vi "5.vi"(2 "逆运动学输入":dbl[](array[numeric])=[0.2, 0.0, 0.3], 3 "123":dbl[](array[numeric]), 4 "机械臂末端姿态":dbl[][](array[numeric])) -> (0 "1235b":dbl[](array[numeric]), 1 "1235a":dbl[](array[numeric]))   [LabVIEW 2014]
uses:
  <vilib>/Utility/file.llb/Read From Spreadsheet File (DBL).vi
panel:
  out "t52":dbl
  out "t6":dbl
  out "t5":dbl
  out "t4":dbl
  out "angle33":dbl
  out "angle32":dbl
  out "angle52":dbl
  out "3角度输出":dbl[](array[numeric])
  out "角度/弧度":dbl
  out "弧度/角度":dbl
  out "az":dbl=1.0
  out "ay":dbl
  out "ax":dbl
  out "angle6":dbl
  out "angle5":dbl
  out "angle4":dbl
  out "angle3":dbl
  out "angle2":dbl
  out "angle1":dbl
  out "逆运动学输出":dbl[](array[numeric])=[0.0, 90.0, 0.0, 0.0, -90.0, -0.0] format="%#.3f"
  in  "机械臂臂长":dbl[](array[numeric])=[558.0, 764.0, 993.0, 420.0]
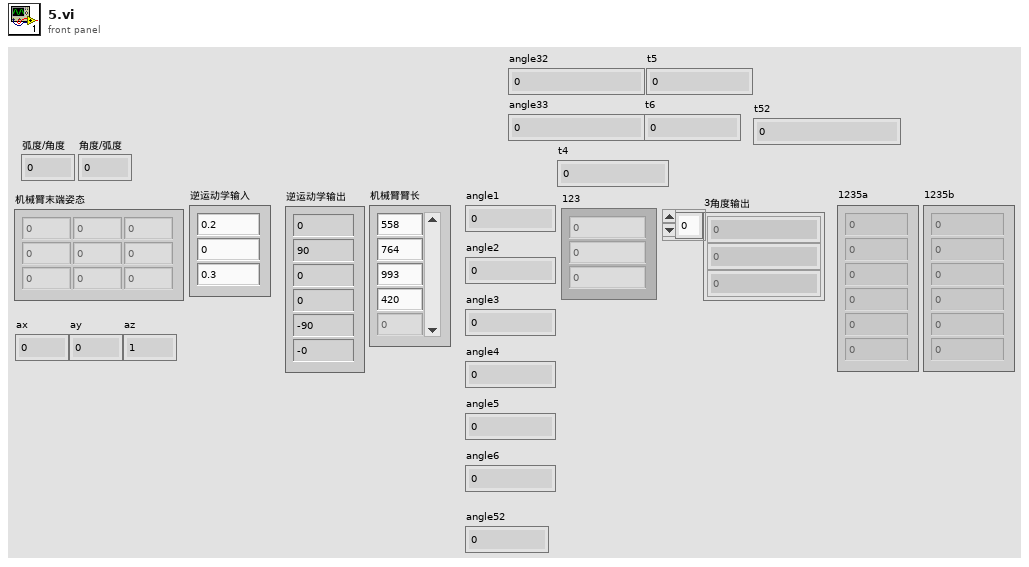
[diagram p1: front panel]
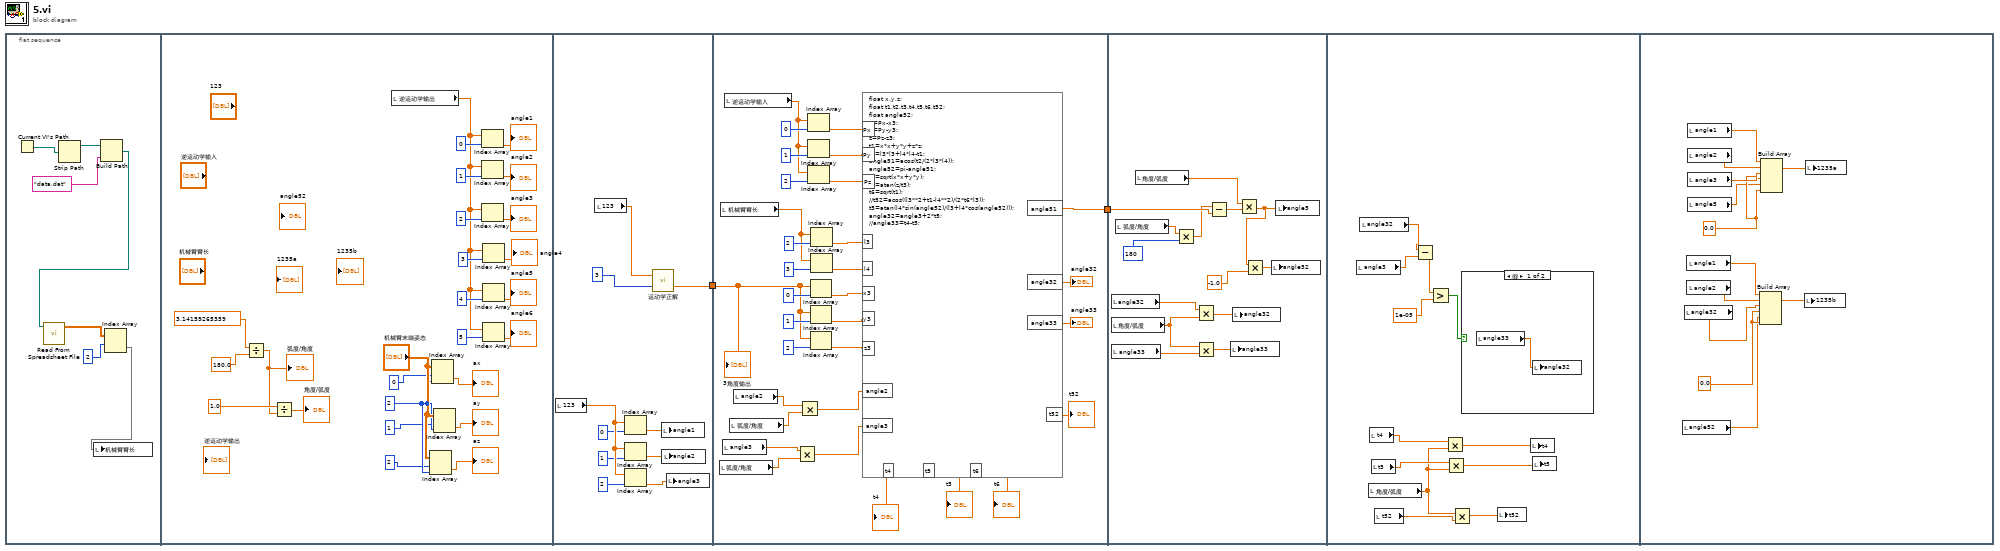
[diagram p0: block diagram]
diagram:
  n1 = flat-sequence {
    tunnel: [w44] -> w1
    tunnel: [w58] -> w2
    tunnel: w1 -> [w70]
    tunnel: w2 -> [w87]
    frame #0 {
      n2 = Current VI's Path() -> (path=w6:path)
      n3 = Strip Path(path=w6) -> (stripped path=w5:path)  [unwired: 1 out]
      n4 = Build Path(base path=w5, name or relative path="data.dat") -> (appended path=w3:path)
      n5 = call-poly <vilib>:"Read From Spreadsheet File.vi"("file path (dialog if empty)"=w3) -> ("all rows"=w9:dbl[][])  [unwired: 6 in, 4 out]
      n6 = Index Array(array=w9, index (row)=2) -> (element=w8:dbl[])  [unwired: 1 in]
      n7 = local write "机械臂臂长"(w8) -> ()
    }
    frame #1 {
      w19 = 2
      n8 = Divide(x=3.14159265359, y=180.0) -> (x/y=w11:dbl)
      "弧度/角度" <- w11
      n9 = Divide(x=1.0, y=w11) -> (x/y=→"角度/弧度":dbl)
      n10 = local read "逆运动学输出"() -> (w23:dbl[])
      n11 = Index Array(array="机械臂末端姿态", index (row)=2, index (col)=w19) -> (element=→"az":dbl)
      n12 = Index Array(array="机械臂末端姿态", index (row)=0, index (col)=w19) -> (element=→"ax":dbl)
      n13 = Index Array(array="机械臂末端姿态", index (row)=1, index (col)=w19) -> (element=→"ay":dbl)
      n14 = Index Array(array=w23, index=0) -> (element=→"angle1":dbl)
      n15 = Index Array(array=w23, index=1) -> (element=→"angle2":dbl)
      n16 = Index Array(array=w23, index=2) -> (element=→"angle3":dbl)
      n17 = Index Array(array=w23, index=3) -> (element=→"angle4":dbl)
      n18 = Index Array(array=w23, index=4) -> (element=→"angle5":dbl)
      n19 = Index Array(array=w23, index=5) -> (element=→"angle6":dbl)
    }
    frame #2 {
      n20 = local read "123"() -> (w39:dbl[])
      n21 = local read "123"() -> (w43:dbl[])
      n22 = Index Array(array=w39, index=0) -> (element=w40:dbl)
      n23 = Index Array(array=w39, index=1) -> (element=w42:dbl)
      n24 = Index Array(array=w39, index=2) -> (element=w41:dbl)
      n25 = call "运动学正解.vi"("正运动学输入"=w43, "关节数"=3) -> ("腕部输出"=w44:dbl[])  [unwired: 2 out]
      n26 = local write "angle1"(w40) -> ()
      n27 = local write "angle2"(w42) -> ()
      n28 = local write "angle3"(w41) -> ()
    }
    frame #3 {
      n29 = local read "弧度/角度"() -> (w47:dbl)
      n30 = local read "机械臂臂长"() -> (w61:dbl[])
      n31 = local read "angle3"() -> (w48:dbl)
      n32 = local read "逆运动学输入"() -> (w74:dbl[])
      n33 = local read "弧度/角度"() -> (w51:dbl)
      n34 = local read "angle2"() -> (w52:dbl)
      n35 = Multiply(x=w48, y=w47) -> (x*y=w46:dbl)
      n36 = Multiply(x=w52, y=w51) -> (x*y=w50:dbl)
      n37 = Index Array(array=w74, index=0) -> (element=w64:dbl)
      n38 = Index Array(array=w74, index=1) -> (element=w65:dbl)
      n39 = Index Array(array=w74, index=2) -> (element=w66:dbl)
      n40 = Index Array(array=w70, index=0) -> (element=w69:dbl)
      n41 = Index Array(array=w70, index=1) -> (element=w68:dbl)
      n42 = Index Array(array=w70, index=2) -> (element=w67:dbl)
      n43 = Index Array(array=w61, index=2) -> (element=w60:dbl)
      n44 = Index Array(array=w61, index=3) -> (element=w59:dbl)
      n45 = formula code="float x,y,z;\nfloat t1,t2,t3,t4,t5,t6,t52;\nfloat angle52;\nx=Px-x3;\ny=Py-y3;\nz=Pz-z3;\nt1=x*x+y*y+z*z;\nt2=l3*l3+l4*l4-t1;\nangle51=acos(t2/(2*l3*l4));\nangle52=pi-angle51;\nt3=sqrt(x*x+y*y);\nt4=atan(z/t3);\nt6=sqrt(t1);\n//t52=acos((l3**2+t1-l4**2)/(2*t6*l3));\nt5=atan(l4*sin(angle52)/(l3+l4*cos(angle52)));\nangle32=angle3+2*t5;\n//angle33=t4-t5;"("Px"=w64, "Py"=w65, "Pz"=w66, "x3"=w69, "y3"=w68, "z3"=w67, "l4"=w59, "l3"=w60, "angle2"=w50, "angle3"=w46) -> ("angle51"=w58:dbl, "angle32"=→"angle32":dbl, "angle33"=→"angle33":dbl, "t4"=→"t4":dbl, "t5"=→"t5":dbl, "t6"=→"t6":dbl, "t52"=→"t52":dbl)
      "3角度输出" <- w70
    }
    frame #4 {
      n46 = local read "angle32"() -> (w82:dbl)
      n47 = local read "角度/弧度"() -> (w79:dbl)
      n48 = local read "angle33"() -> (w80:dbl)
      n49 = local read "弧度/角度"() -> (w91:dbl)
      n50 = local read "角度/弧度"() -> (w88:dbl)
      n51 = Multiply(x=w91, y=180) -> (x*y=w86:dbl)
      n52 = Multiply(x=w82, y=w79) -> (x*y=w81:dbl)
      n53 = Multiply(x=w79, y=w80) -> (x*y=w78:dbl)
      n54 = Subtract(x=w86, y=w87) -> (x-y=w89:dbl)
      n55 = local write "angle33"(w78) -> ()
      n56 = local write "angle32"(w81) -> ()
      n57 = Multiply(x=w88, y=w89) -> (x*y=w84:dbl)
      n58 = Multiply(x=w84, y=-1.0) -> (x*y=w83:dbl)
      n59 = local write "angle52"(w83) -> ()
      n60 = local write "angle5"(w84) -> ()
    }
    frame #5 {
      n61 = local read "angle3"() -> (w102:dbl)
      n62 = local read "angle32"() -> (w103:dbl)
      n63 = local read "角度/弧度"() -> (w93:dbl)
      n64 = local read "t4"() -> (w98:dbl)
      n65 = local read "t5"() -> (w96:dbl)
      n66 = local read "t52"() -> (w94:dbl)
      n67 = Subtract(x=w103, y=w102) -> (x-y=w101:dbl)
      n68 = Greater?(x=w101, y=1e-05) -> (0:w99:bool)
      n69 = Multiply(x=w98, y=w93) -> (x*y=w97:dbl)
      n70 = Multiply(x=w96, y=w93) -> (x*y=w95:dbl)
      n71 = Multiply(x=w93, y=w94) -> (x*y=w92:dbl)
      n72 = case shown="假" w99 {
        frame False {
          n73 = local read "angle33"() -> (w104:dbl)
          n74 = local write "angle32"(w104) -> ()
        }
        frame True {
        }
      }
      n75 = local write "t52"(w92) -> ()
      n76 = local write "t4"(w97) -> ()
      n77 = local write "t5"(w95) -> ()
    }
    frame #6 {
      w107 = 0.0
      w109 = 0.0
      n78 = local read "angle52"() -> (w108:dbl)
      n79 = local read "angle32"() -> (w105:dbl)
      n80 = local read "angle1"() -> (w110:dbl)
      n81 = local read "angle2"() -> (w111:dbl)
      n82 = local read "angle1"() -> (w116:dbl)
      n83 = local read "angle2"() -> (w115:dbl)
      n84 = local read "angle3"() -> (w114:dbl)
      n85 = local read "angle5"() -> (w106:dbl)
      n86 = Build Array(w110, w111, w105, w109, w108, w109) -> (w112:dbl[])
      n87 = Build Array(w116, w115, w114, w107, w106, w107) -> (w113:dbl[])
      n88 = local write "1235b"(w112) -> ()
      n89 = local write "1235a"(w113) -> ()
    }
  }
